vi "Read HistorianPath.vi"(8 "error in (no error)":errorcluster, 11 "DBAL-BIN in":refnum<class "DBAL-BIN.lvclass">) -> (0 "error out":errorcluster, 2 "HistorianPath":path, 3 "DBAL-BIN out":refnum<class "DBAL-BIN.lvclass">)   [LabVIEW 2020, in "DBAL-BIN.lvclass"]
uses:
  DBAL-BIN.lvclass
  DBAL-BIN.lvclass/DBAL-BIN.ctl
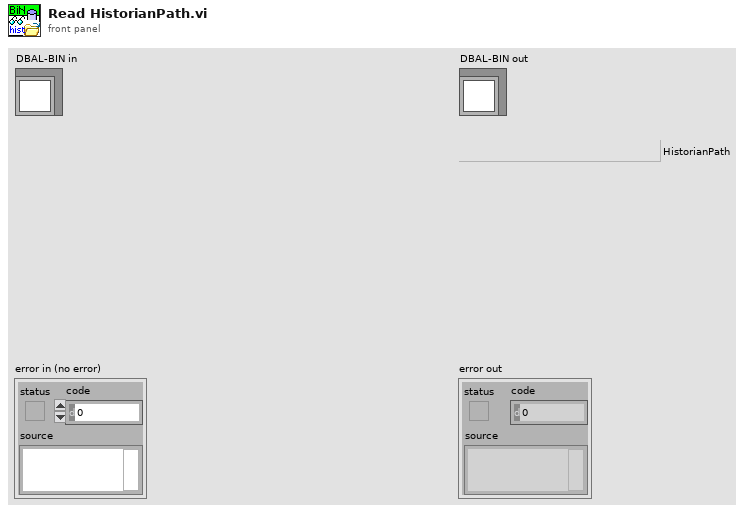
[diagram p1: front panel]
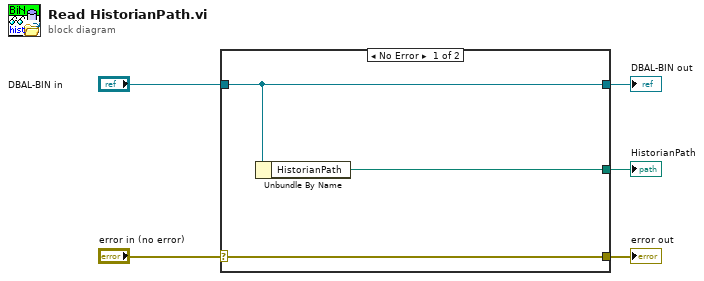
[diagram p0: block diagram]
diagram:
  n1 = case shown="No Error" "error in (no error)" {
    selector: "error in (no error)" -> [w8 w9]
    tunnel: [w8 w9] -> w4
    tunnel: [w7 w10] -> w2
    tunnel: "DBAL-BIN in" -> [w7 w10]
    tunnel: [w6 _] -> w1
    frame No Error {
      n2 = Unbundle By Name(w7) -> ("HistorianPath"=w6:path)
    }
    frame Error {
    }
  }
  "error out" <- w4
  "DBAL-BIN out" <- w2
  "HistorianPath" <- w1
